vi "Autocorrelation_ph.vi"(0 "X":dbl[](array[numeric]) format="%.2f", 3 "Autocorrelation of X":dbl[](array[numeric]) format="%.4f", 4 "Block No":i32=1) -> (6 "Autocorrelation of X":dbl[](array[numeric]) format="%.4f")   [LabVIEW 2011]
uses:
  <vilib>/Analysis/2dsp.llb/1D Auto Correlation (DBL).vi
  <vilib>/Analysis/NI_AALBase.lvlib
  <vilib>/Analysis/NI_AALPro.lvlib
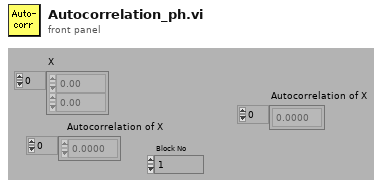
[diagram p1: front panel]
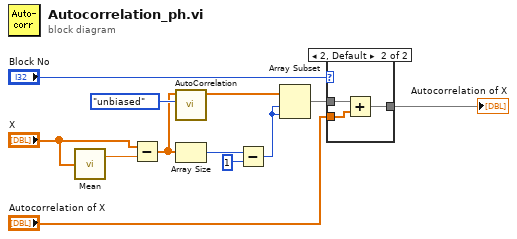
[diagram p0: block diagram]
diagram:
  n1 = call <vilib>:"Mean.vi"("X"="X") -> ("mean"=w10:dbl)  [unwired: 1 out]
  n2 = Subtract(x="X", y=w10) -> (x-y=w4:dbl[])
  n3 = call-poly <vilib>:"AutoCorrelation.vi"("normalization"=enum32{"none", "unbiased", "biased"}."unbiased", "X"=w4) -> ("Rxx"=w3:dbl[])  [unwired: 9 out]
  n4 = Array Size(array=w4) -> (size(s)=w11:i32)
  n5 = Subtract(x=w11, y=1) -> (x-y=w2:i32)
  n6 = Array Subset(array=w3, index=w2, length=w2) -> (w1:dbl[])
  n7 = case shown="2, Default" "Block No" {
    tunnel: [w13 w16] -> w7
    tunnel: w1 -> [w13 w15]
    tunnel: "Autocorrelation of X" -> [_ w14]
    frame 1 {
    }
    frame 2, Default {
      n8 = Add(x=w15, y=w14) -> (x+y=w16:dbl[])
    }
  }
  "Autocorrelation of X" <- w7
